vi "Autonomous.vi"   [LabVIEW 2017]
doc: "This VI starts when autonomous period begins, and will automatically be terminated when it ends. You can carry out timed or sensor driven operations directly to I/O or to subsystems without needing to return to the caller."
uses:
  <vilib>/Rock Robotics/Network Tables/NT Read String.vi
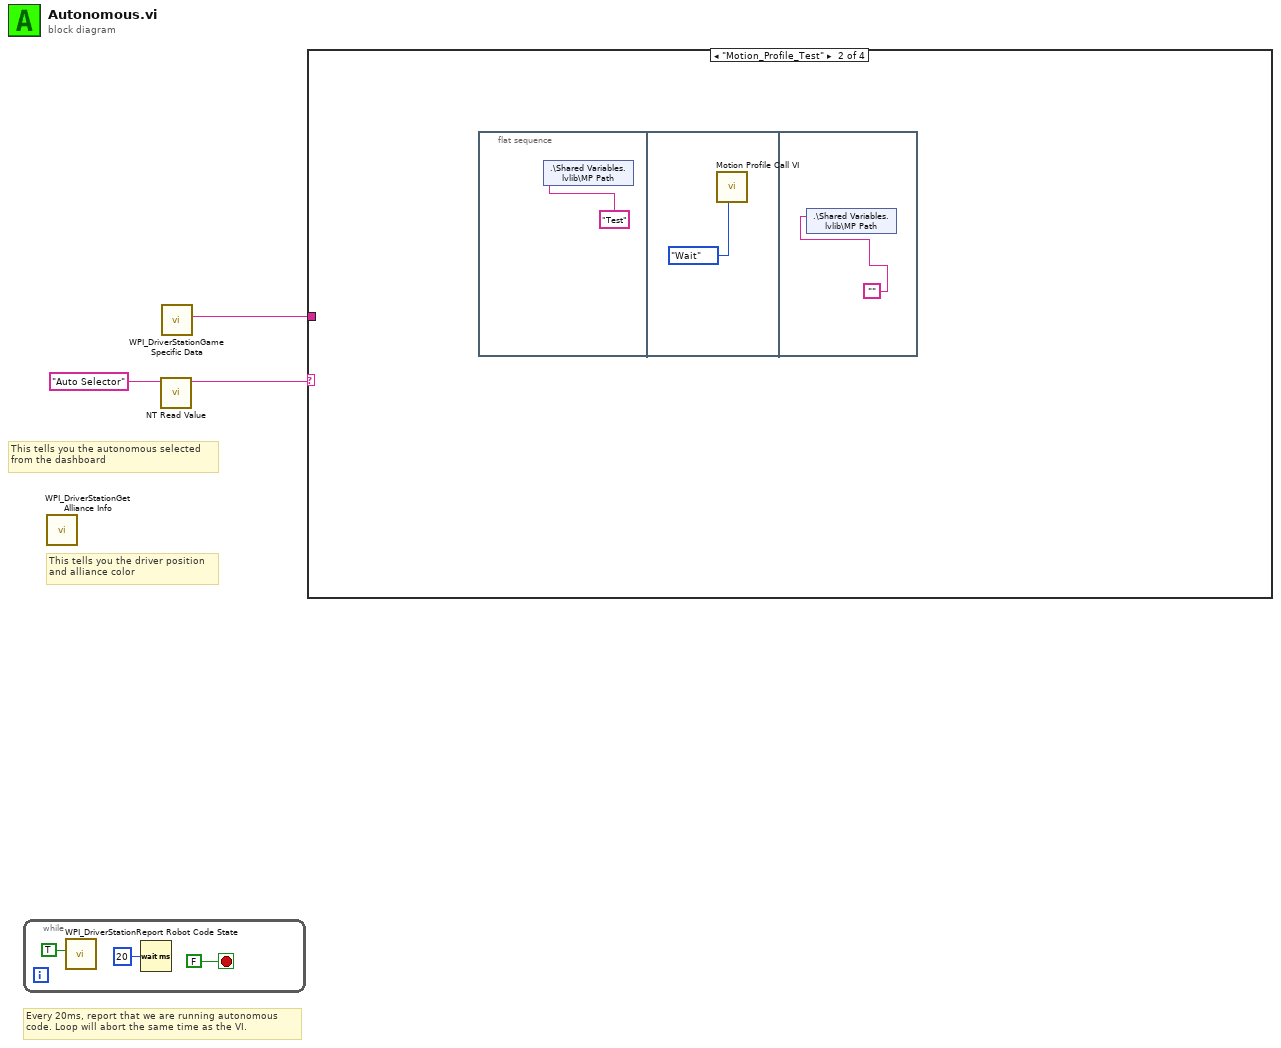
[diagram p0: block diagram]
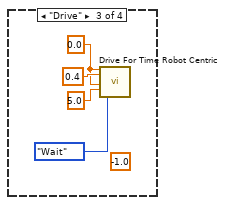
[diagram p3: hidden frame]
diagram:
  # "This tells you the autonomous selected\nfrom the dashboard"
  # "Every 20ms, report that we are running autonomous\ncode. Loop will abort the same time as the VI."
  # "This tells you the driver position\nand alliance color"
  n1 = while {
    stop <- FALSE stop-if-true
    n2 = call <vilib>:"WPI_DriverStationReport Robot Code State.vi"("Autonomous"=TRUE) -> ()  [unwired: 10 in, 1 out]
    n3 = Wait (ms)(milliseconds to wait=u32 20) -> ()  [unwired: 1 out]
  }
  n4 = call <vilib>:"WPI_DriverStationGet Alliance Info.vi"() -> ()  [unwired: 12 out]
  n5 = call-poly <vilib>:"NT Read Value.vi"("Name"="Auto Selector") -> ("String"=w2:string)  [unwired: 9 in, 1 out]
  n6 = call <vilib>:"WPI_DriverStationGame Specific Data.vi"() -> ("Game Specific Data"=w1:string)  [unwired: 11 in]
  n7 = case shown="\"Motion_Profile_Test\"" w2 {
    tunnel: w1 -> [_ _ _ _]
    frame Default {
      # "You can put your main auto here, or you can right-click on the case and make any\nother frame be the default case."
      # "This is the frame that will execute if no selection is made, or if it is not recognized"
    }
    frame "Motion_Profile_Test" {
      n8 = flat-sequence {
        frame #0 {
          n9 = shared-variable ".\\Shared Variables.lvlib\\MP Path"("Test" ("MP Path")) -> ()  [unwired: 1 in, 1 out]
        }
        frame #1 {
          n10 = call "Motion Profile Call VI.vi"("Synchronication"=enum16{"Start", "Wait"}."Wait") -> ()  [unwired: 10 in, 1 out]
        }
        frame #2 {
          n11 = shared-variable ".\\Shared Variables.lvlib\\MP Path"("") -> ()  [unwired: 1 in, 1 out]
        }
      }
    }
    frame "Drive" {
      (unwired) -1.0 ("Distance From Peg (inches)")
      w10 = 0.0 ("Left/right")
      n12 = call "Drive For Time Robot Centric.vi"("Left/right"=w10, "Forward/Backwards"=0.4, "Rotation"=w10, "Seconds"=5.0, "Synchronization"=enum16{"Start", "Wait"}."Wait") -> ()  [unwired: 13 in, 2 out]
    }
    frame "Test" {
    }
  }
